vi "ad analog in.vi"(7 "data":sgl, 8 "error in (no error)":errorcluster, 9 "range":i32, 10 "cha":i32, 11 "adh":i32) -> (0 "error out":errorcluster, 3 "function return":i32, 5 "data out":sgl)   [LabVIEW 2021, in "libad4.lvlib"]
doc: "LIBAD4 function: ad_analog_in (int32_t adh, int32_t cha, int32_t range, float *data);\n\nHelper function for ad_discrete_in. Allows analog channels to be addressed directly and automatically converts the discrete values to float."
uses:
  <userlib>/libad4/libad4.lvlib
  <userlib>/libad4/libad4.dll
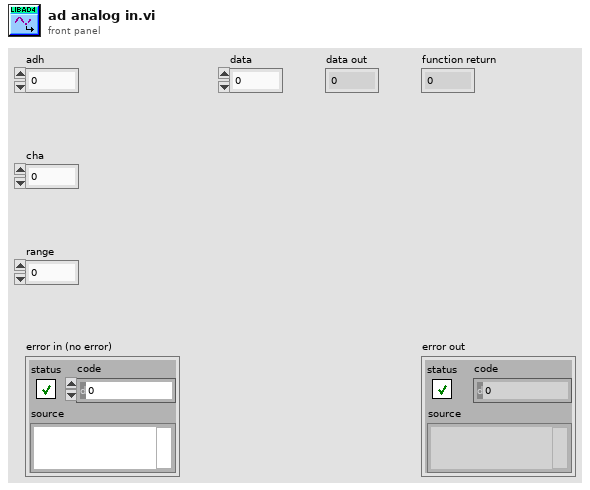
[diagram p1: front panel]
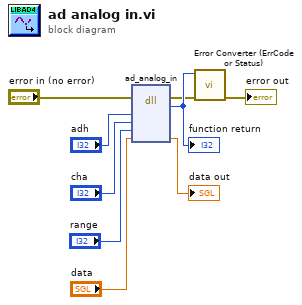
[diagram p0: block diagram]
diagram:
  n1 = dll-call lib="C:/Program Files/National Instruments/LabVIEW 2021/user.lib/libad4/libad4.*" fn="ad_analog_in"(error in="error in (no error)", "adh"="adh", "cha"="cha", "range"="range", "data"="data") -> (error out=w2:errorcluster, "return type"=w9:i32, "data"=→"data out":sgl)  [unwired: 5 in, 1 out]
  "function return" <- w9
  n2 = call <userlib>:"Error Converter (ErrCode or Status).vi"("error in (no error)"=w2, "error code"=w9) -> ("error out"=→"error out":errorcluster)  [unwired: 9 in]
